vi "Convertpourcent2.vi"() -> ()   [LabVIEW 2015]
panel:
  in  "input variable":i16
  out "output variable":u8
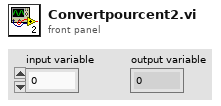
[diagram p1: front panel]
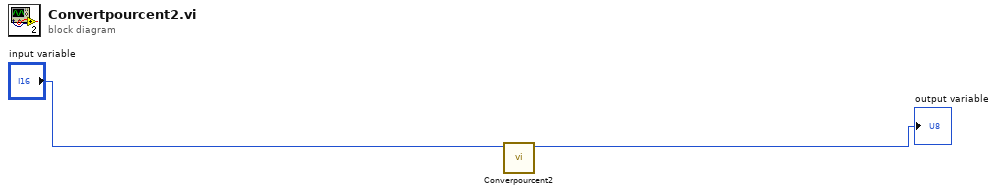
[diagram p0: block diagram]
diagram:
  n1 = call "Converpourcent2.vi"("input variable"="input variable") -> ("output variable"=→"output variable":u8)  [unwired: 10 in]
